vi "test_image_avg_no_reshape.vi"() -> ()   [LabVIEW 2013]
panel:
  out "Numeric":i32
  in  "average in other dim":dbl
  in  "points / pixel":i32
  out "output array":dbl[][](array[numeric])
  in  "stop":bool
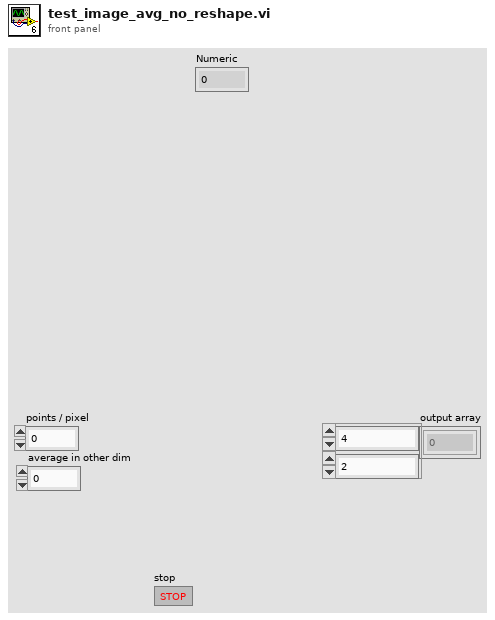
[diagram p1: front panel]
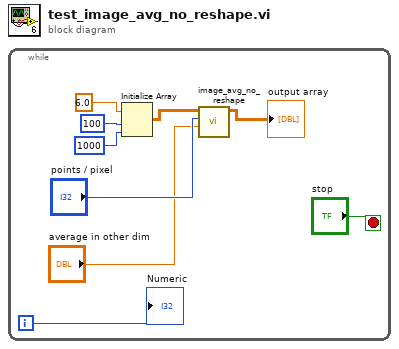
[diagram p0: block diagram]
diagram:
  n1 = while {
    i -> [w1]
    stop <- "stop" stop-if-true
    n2 = Initialize Array(6.0 ("element"), 100 ("dimension size"), 1000 ("dimension size")) -> (w6:dbl[][])
    n3 = call "image_avg_no_reshape.vi"("Numeric"="average in other dim", "points / pixel"="points / pixel", "input array"=w6) -> ("output array"=→"output array":dbl[][])  [unwired: 8 in]
    "Numeric" <- w1
  }
